vi "Show Tips.vi"(8 "error in (no error)":errorcluster caption="错误输入（无错误）", 9 "显示内容":string, 10 "是否清空":bool, 11 "LstBox句柄输入":refnum<vi>) -> (0 "error out":errorcluster caption="错误输出", 3 "LstBox句柄输出":refnum<vi>)   [LabVIEW 2017]
panel:
  out "数组":string[](array[string])
  out "当前状态":i32(listbox)
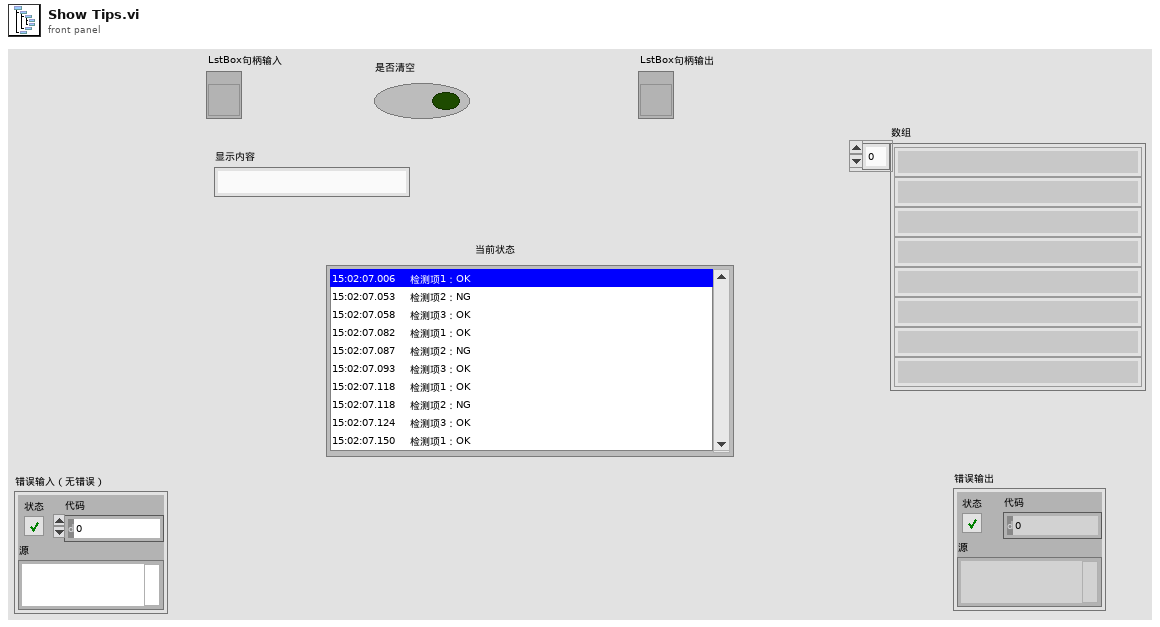
[diagram p1: front panel]
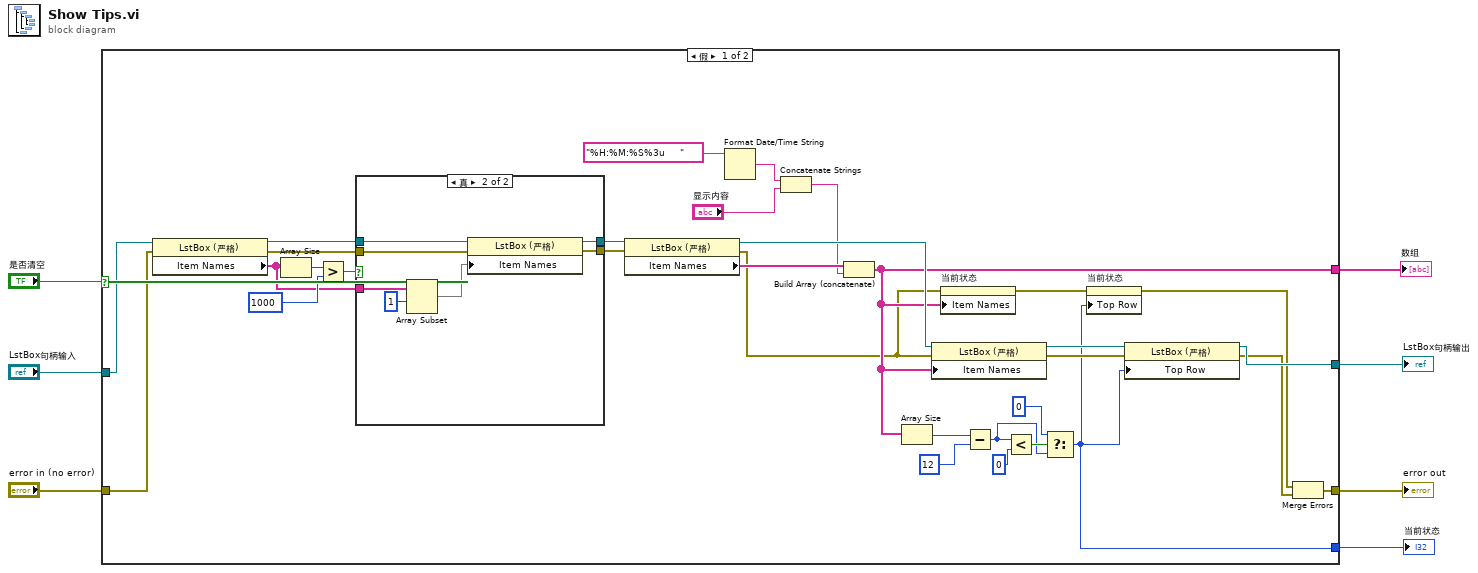
[diagram p0: block diagram]
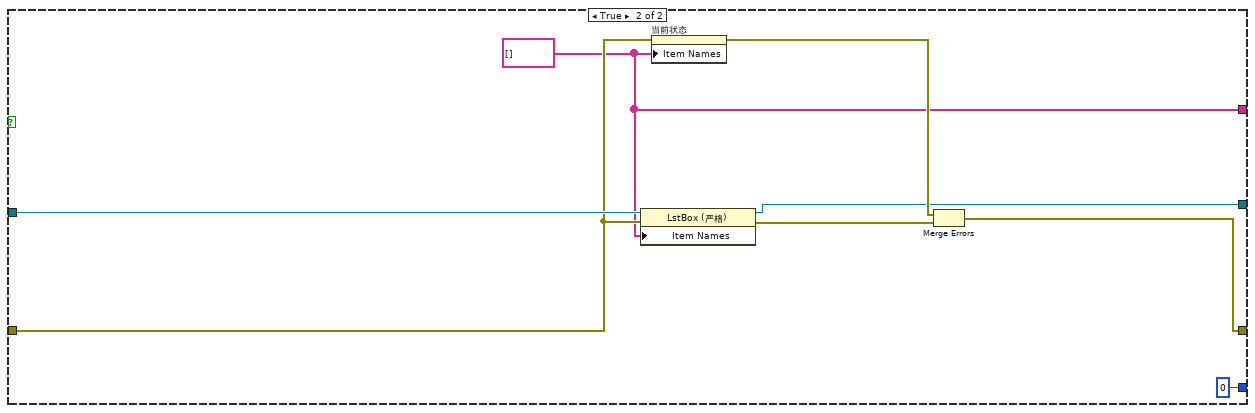
[diagram p3: hidden frame]
diagram:
  n1 = case shown="假" "是否清空" {
    tunnel: "LstBox句柄输入" -> [w39 w56]
    tunnel: "error in (no error)" -> [w11 w55]
    tunnel: [w36 w52] -> w4
    tunnel: [w28 w51] -> w1
    tunnel: [w31 w50] -> w3
    tunnel: [w23 0] -> w2
    frame False {
      n2 = property class="LstBox (严格)"(reference=w39, error in=w11) -> (reference out=w13:refnum<vi>, error out=w10:errorcluster, "Item Names"=w8:string[])
      n3 = Array Size(array=w8) -> (size(s)=w16:i32)
      n4 = Greater?(x=w16, y=1000) -> (0:w14:bool)
      n5 = case shown="真" w14 {
        tunnel: w13 -> [w41 w48]
        tunnel: [w41 w47] -> w12
        tunnel: w10 -> [w40 w46]
        tunnel: [w40 w45] -> w9
        tunnel: w8 -> [_ w44]
        frame False {
        }
        frame True {
          n6 = Array Subset(array=w44, index=1 ("索引")) -> (w42:string[])  [unwired: 1 in]
          n7 = property class="LstBox (严格)"(reference=w48, error in=w46, "Item Names"=w42) -> (reference out=w47:refnum<vi>, error out=w45:errorcluster)
        }
      }
      n8 = property class="LstBox (严格)"(reference=w12, error in=w9) -> (reference out=w37:refnum<vi>, error out=w30:errorcluster, "Item Names"=w38:string[])
      n9 = Format Date/Time String(time format string (%c)="%H:%M:%S%3u     " ("时间格式字符串(%c)")) -> (date/time string=w19:string)  [unwired: 2 in]
      n10 = Concatenate Strings(w19, "显示内容") -> (w17:string)
      n11 = Build Array (concatenate)(w38, w17) -> (w31:string[])
      n12 = Array Size(array=w31) -> (size(s)=w33:i32)
      n13 = property class="LstBox (严格)"(reference=w37, error in=w30, "Item Names"=w31) -> (reference out=w35:refnum<vi>, error out=w34:errorcluster)
      n14 = property on="当前状态" class="LstBox (严格)"(error in=w30, "Item Names"=w31) -> (error out=w29:errorcluster)  [unwired: 1 in, 1 out]
      n15 = Subtract(x=w33, y=12) -> (x-y=w22:i32)
      n16 = Less?(x=w22, y=0) -> (x < y?=w24:bool)
      n17 = Select(t=0, s=w24, f=w22) -> (s? t:f=w23:i32)
      n18 = property on="当前状态" class="LstBox (严格)"(error in=w29, "Top Row"=w23) -> (error out=w26:errorcluster)  [unwired: 1 in, 1 out]
      n19 = property class="LstBox (严格)"(reference=w35, error in=w34, "Top Row"=w23) -> (reference out=w36:refnum<vi>, error out=w27:errorcluster)
      n20 = Merge Errors(w26, w27) -> (w28:errorcluster)
    }
    frame True {
      w50 = string[] [] ("项名")
      n21 = property class="LstBox (严格)"(reference=w56, error in=w55, "Item Names"=w50) -> (reference out=w52:refnum<vi>, error out=w53:errorcluster)
      n22 = property on="当前状态" class="LstBox (严格)"(error in=w55, "Item Names"=w50) -> (error out=w54:errorcluster)  [unwired: 1 in, 1 out]
      n23 = Merge Errors(w54, w53) -> (w51:errorcluster)
    }
  }
  "当前状态" <- w2
  "error out" <- w1
  "LstBox句柄输出" <- w4
  "数组" <- w3
